vi "Get Plot at Mouse Click in Plot Area [ACCA].vi"(8 "error in (no error)":errorcluster, 10 "Mouse Click Coordinates":T1, 11 "XY Graph":refnum<vi>) -> (0 "error out":errorcluster, 1 "Plot Index":i32, 3 "XY Graph":refnum<vi>)   [LabVIEW 2021, in "Graphs.lvlib"]
uses:
  Graphs.lvlib
  <vilib>/Utility/miscctls.llb/LVPoint32TypeDef.ctl
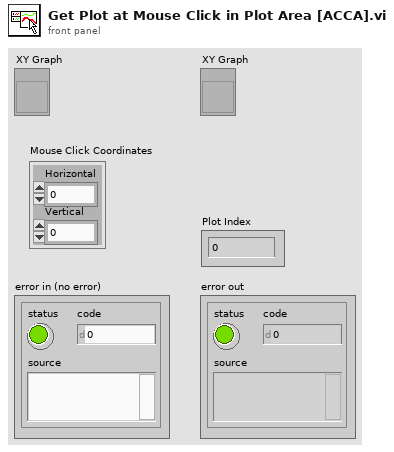
[diagram p1: front panel]
types:
  T1 = typedef "LVPoint32TypeDef.ctl" = cluster{"Horizontal":i32, "Vertical":i32}
  T2 = typedef "LVRectTypeDef.ctl" = cluster{"Left":i16, "Top":i16, "Right":i16, "Bottom":i16}
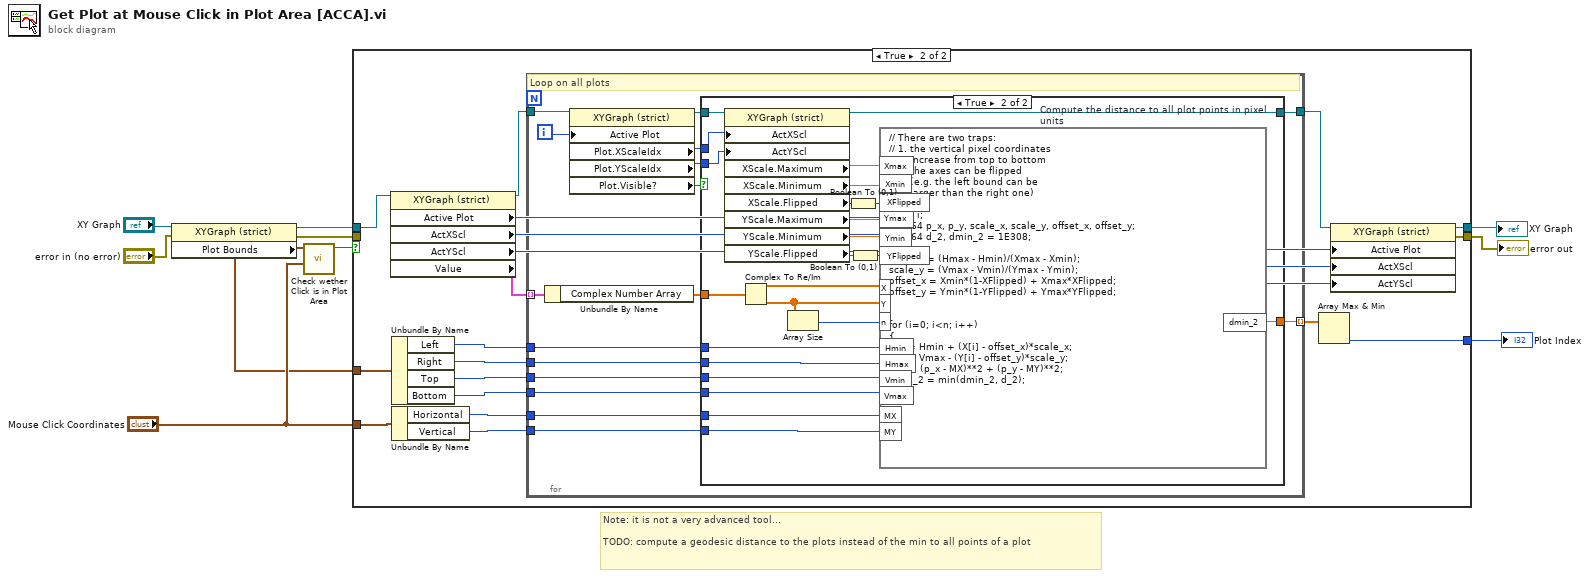
[diagram p0: block diagram]
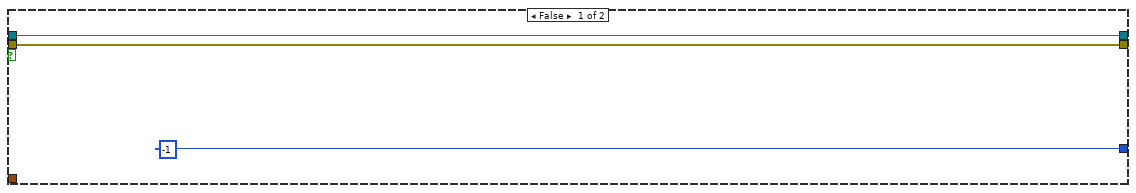
[diagram p2: hidden frame]
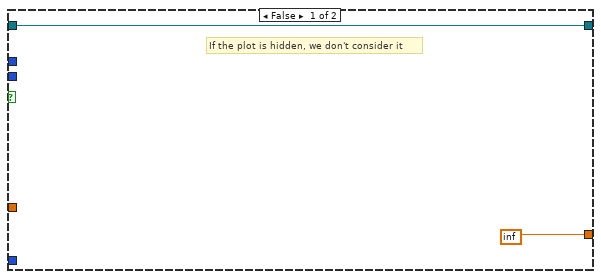
[diagram p3: hidden frame]
diagram:
  # "Note: it is not a very advanced tool...\n\nTODO: compute a geodesic distance to the plots instead of the min to all points of a plot"
  n1 = property class="XYGraph (strict)"(reference="XY Graph", error in="error in (no error)") -> (reference out=w6:refnum<vi>, error out=w7:errorcluster, "Plot Bounds"=w2:T2)
  n2 = call "Check wether Click is in Plot Area.vi"("Mouse Click Coordinates"="Mouse Click Coordinates", "Plot Bounds"=w2) -> ("Is in Plot Area?"=w8:bool)  [unwired: 8 in, 1 out]
  n3 = case shown="True" w8 {
    tunnel: w7 -> [w12 _]
    tunnel: w6 -> [w13 w32]
    tunnel: [w13 w31] -> w1
    tunnel: [w12 w30] -> w5
    tunnel: [-1 ("Plot Index") w27] -> w4
    tunnel: "Mouse Click Coordinates" -> [_ w29]
    tunnel: w2 -> [_ w28]
    frame False {
    }
    frame True {
      n4 = property class="XYGraph (strict)"(reference=w32) -> (reference out=w26:refnum<vi>, "Active Plot"=w24:u32, "ActXScl"=w23:i32, "ActYScl"=w22:i32, "Value"=w14:cluster{"Complex Number Array":cdb[]}[])  [unwired: 1 in, 1 out]
      n5 = Unbundle By Name(w28) -> ("Left"=w21:i16, "Right"=w20:i16, "Top"=w19:i16, "Bottom"=w18:i16)
      n6 = Unbundle By Name(w29) -> ("Horizontal"=w17:i32, "Vertical"=w16:i32)
      n7 = for {
        tunnel: w14 -> [w48] mode=indexing
        tunnel: w26 -> [w35]
        tunnel: [w43] -> w25
        tunnel: w21 -> [w42]
        tunnel: w20 -> [w41]
        tunnel: w19 -> [w40]
        tunnel: w18 -> [w39]
        tunnel: w17 -> [w38]
        tunnel: w16 -> [w37]
        tunnel: [w36] -> w15 mode=indexing
        i -> [w47]
        # "Loop on all plots"
        n8 = Unbundle By Name(w48) -> ("Complex Number Array"=w33:cdb[])
        n9 = property class="XYGraph (strict)"(reference=w35, "Active Plot"=w47) -> (reference out=w46:refnum<vi>, "Plot.XScaleIdx"=w45:u32, "Plot.YScaleIdx"=w44:u32, "Plot.Visible?"=w34:bool)  [unwired: 1 in, 1 out]
        n10 = case shown="True" w34 {
          tunnel: w33 -> [_ w53]
          tunnel: w46 -> [w50 w73]
          tunnel: w45 -> [_ w72]
          tunnel: w44 -> [_ w71]
          tunnel: [w50 w70] -> w43
          tunnel: w42 -> [_ w65]
          tunnel: w41 -> [_ w64]
          tunnel: w40 -> [_ w63]
          tunnel: w39 -> [_ w62]
          tunnel: w38 -> [_ w61]
          tunnel: w37 -> [_ w60]
          tunnel: [inf w59] -> w36
          frame False {
            # "If the plot is hidden, we don't consider it"
          }
          frame True {
            n11 = property class="XYGraph (strict)"(reference=w73, "ActXScl"=w72, "ActYScl"=w71) -> (reference out=w70:refnum<vi>, "XScale.Maximum"=w69:dbl, "XScale.Minimum"=w68:dbl, "XScale.Flipped"=w58:bool, "YScale.Maximum"=w67:dbl, "YScale.Minimum"=w66:dbl, "YScale.Flipped"=w56:bool)  [unwired: 1 in, 1 out]
            n12 = Complex To Re/Im(x + iy=w53) -> (x=w52:dbl[], y=w51:dbl[])
            n13 = Array Size(array=w51) -> (size(s)=w54:i32)
            n14 = Boolean To (0,1)(Boolean=w58) -> (0, 1=w57:i16)
            n15 = Boolean To (0,1)(Boolean=w56) -> (0, 1=w55:i16)
            n16 = formula code="// There are two traps:\n// 1. the vertical pixel coordinates\n//     increase from top to bottom\n// 2. the axes can be flipped\n//     (e.g. the left bound can be\n//     larger than the right one)\n\nint32 i;\nfloat64 p_x, p_y, scale_x, scale_y, offset_x, offset_y;\nfloat64 d_2, dmin_2 = 1E308;\n\nscale_x = (Hmax - Hmin)/(Xmax - Xmin);\nscale_y = (Vmax - Vmin)/(Ymax - Ymin);\noffset_x = Xmin*(1-XFlipped) + Xmax*XFlipped;\noffset_y = Ymin*(1-YFlipped) + Ymax*YFlipped;\n\n\nfor (i=0; i<n; i++)\n{\np_x = Hmin + (X[i] - offset_x)*scale_x;\np_y = Vmax - (Y[i] - offset_y)*scale_y;\nd_2 = (p_x - MX)**2 + (p_y - MY)**2;\ndmin_2 = min(dmin_2, d_2);\n}" "Compute the distance to all plot points in pixel units"("Xmax"=w69, "Xmin"=w68, "Ymax"=w67, "Ymin"=w66, "Hmin"=w65, "Hmax"=w64, "Vmin"=w63, "Vmax"=w62, "MX"=w61, "MY"=w60, "X"=w52, "Y"=w51, "XFlipped"=w57, "YFlipped"=w55, "n"=w54) -> ("dmin_2"=w59:dbl)
          }
        }
      }
      n17 = Array Max & Min(array=w15) -> (min index (indices)=w27:i32)  [unwired: 3 out]
      n18 = property class="XYGraph (strict)"(reference=w25, "Active Plot"=w24, "ActXScl"=w23, "ActYScl"=w22) -> (reference out=w31:refnum<vi>, error out=w30:errorcluster)  [unwired: 1 in]
    }
  }
  "Plot Index" <- w4
  "XY Graph" <- w1
  "error out" <- w5
